vi "Get Min.vi"(8 "error in (no error)":errorcluster, 11 "Range in":refnum<class "Range.lvclass">) -> (0 "error out":errorcluster, 2 "Min":u64, 3 "Range out":refnum<class "Range.lvclass">)   [LabVIEW 2020, in "Range.lvclass"]
uses:
  Range.lvclass
  Range.lvclass/Range.ctl
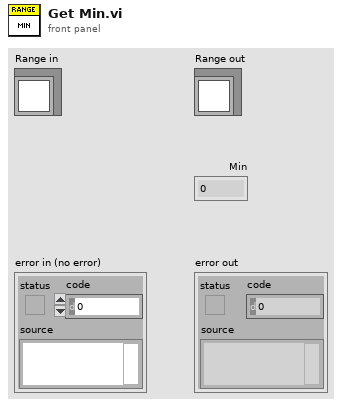
[diagram p1: front panel]
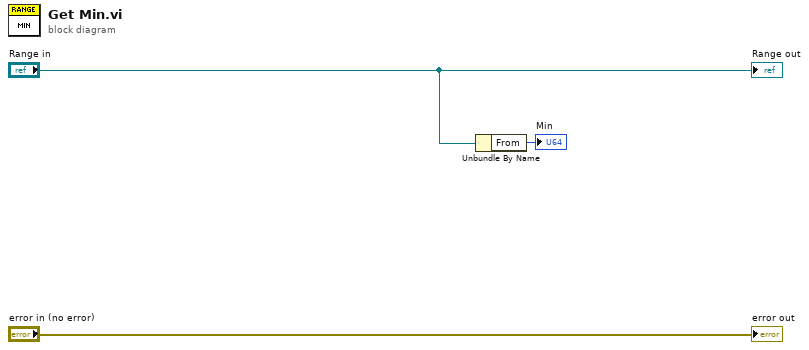
[diagram p0: block diagram]
diagram:
  n1 = Unbundle By Name("Range in") -> ("From"=→"Min":u64)
  "error out" <- "error in (no error)"
  "Range out" <- "Range in"
